vi "Check CRC.vi"(8 "error in (no error)":errorcluster, 10 "IP":i16, 11 "Refnum in":refnum<k21>) -> (0 "error out":errorcluster, 2 "Numeric":i16, 3 "Button":bool)   [LabVIEW 2018, in "Modbus_Processing_Unit.lvlib" / "MPU.lvclass"]
uses:
  MPU.lvclass
  <vilib>/rvi/DataTransferAndStorage/Container/Common/niFpgaContainerExecOnDevCompGetState.vi
  <vilib>/rvi/Emulation/niFpgaEmulationIsFPGAContextNoSignature.vi
  <vilib>/rvi/DataTransferAndStorage/Container/Common/niFpgaContainerGetUniqueNameForEmu.vi
  <vilib>/rvi/Emulation/niFpgaProcessEmulError.vi
  <vilib>/rvi/Emulation/niFpgaSctlEmulationGetInTimedLoop.vi
  <vilib>/rvi/errors/nirviReportUnexpectedCaseInternalError (U32).vi
  <vilib>/rvi/Memory/Memory_Emulation/niFpgaMemoryEmulationCacheClearOnFirstRun.vi
  <vilib>/rvi/Memory/Memory_Emulation/nirvimemoryEmulationManagerCache_MakeExclusive.vi
  <vilib>/rvi/Memory/Memory_Emulation/niFpgaMemoryEmulationValidateCache.vi
  <vilib>/rvi/Memory/Memory_Emulation/nirvimemoryEmulationManagerCache_InsertValue.vi
  <vilib>/Utility/error.llb/Clear Errors.vi
  <vilib>/rvi/Memory/Memory_Emulation/nirvimemoryEmulationManagerCache_ReleaseExclusive.vi
  <vilib>/rvi/Memory/Memory_Emulation/nirvimemoryEmulationManagerCache_GetValue.vi
  <vilib>/rvi/Memory/Memory_Emulation/nirvimemoryEmulationManagerCache_SetValue.vi
  <vilib>/rvi/Emulation/niFpgaSctlEmulationResourceMgr.vi
  <vilib>/rvi/DataTransferAndStorage/Container/XNode/niFpgaContainer.xnode
  <vilib>/rvi/Memory/Memory_Emulation/niFpgaMemoryEmulationRefIn.vi
  Modbus_Processing_Unit.lvlib
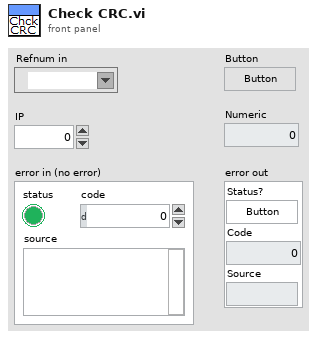
[diagram p1: front panel]
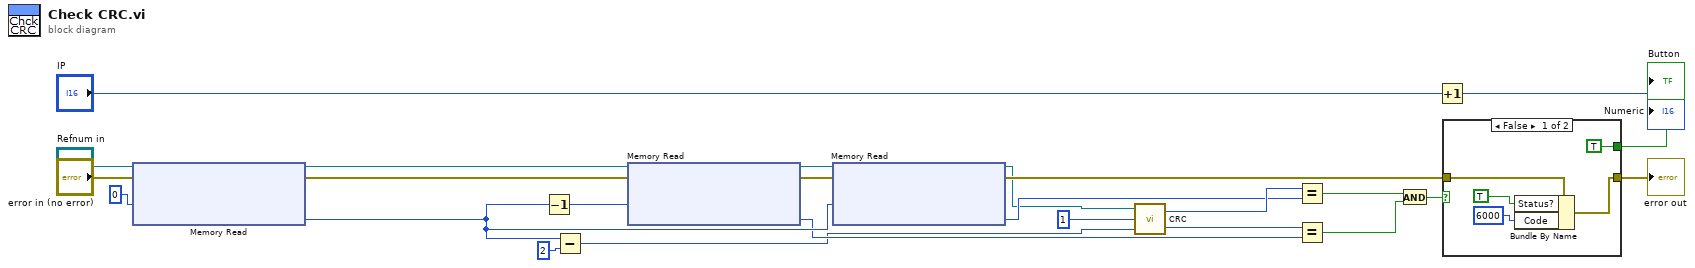
[diagram p0: block diagram]
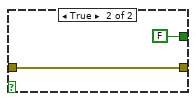
[diagram p2: hidden frame]
diagram:
  n1 = xnode ("Memory Read")("Address"=u32 0, "error in (no error)"="error in (no error)", "Memory In"="Refnum in") -> ("Data"=w23:u8, "error out"=w16:errorcluster, "Memory Out"=w11:refnum<k21>)
  n2 = Decrement(x=w23) -> (x-1=w20:u8)
  n3 = Subtract(x=w23, y=2) -> (x-y=w19:i32)
  n4 = xnode ("Memory Read")("Address"=w20, "error in (no error)"=w16, "Memory In"=w11) -> ("Data"=w22:u8, "error out"=w17:errorcluster, "Memory Out"=w14:refnum<k21>)
  n5 = xnode ("Memory Read")("Address"=w23, "error in (no error)"=w17, "Memory In"=w14) -> ("Data"=w21:u8, "error out"=w18:errorcluster, "Memory Out"=w15:refnum<k21>)
  n6 = call "CRC.vi"("Size"=w19, "Offset"=i16 1, "Data"=w15) -> ("CRC Lo"=w24:u8, "CRC Hi"=w25:u8)
  n7 = Equal?(x=w25, y=w21) -> (x = y?=w5:bool)
  n8 = Equal?(x=w24, y=w22) -> (x = y?=w6:bool)
  n9 = And(x=w5, y=w6) -> (x .and. y?=w4:bool)
  n10 = Increment(x="IP") -> (x+1=→"Numeric":i16)
  n11 = case shown="False" w4 {
    tunnel: w18 -> [w30 w32]
    tunnel: [w29 w32] -> w7
    tunnel: [TRUE FALSE] -> w8
    frame False {
      n12 = Bundle By Name(cluster=w30, "Status?"=TRUE, "Code"=6000) -> (w29:errorcluster)
    }
    frame True {
    }
  }
  "Button" <- w8
  "error out" <- w7
